vi "Recreate Client.vi"(8 "error in":errorcluster, 10 "cluster id":string, 11 "grpc client id in":T1) -> (0 "error out":errorcluster, 3 "grpc client id out":T1)   [LabVIEW 2020, in "Measurement Plugin Session Management V1.lvlib" / "Session Reservation.lvclass"]
uses:
  Session Reservation.lvclass
  <vilib>/gRPC/LabVIEW gRPC Library/Shared/grpcId.ctl
  Generated/Measurement Plugin Session Management Client/MeasurementLink Session Management Client.lvlib
  <vilib>/gRPC/LabVIEW gRPC Library/grpc-lvsupport-release.lvlib
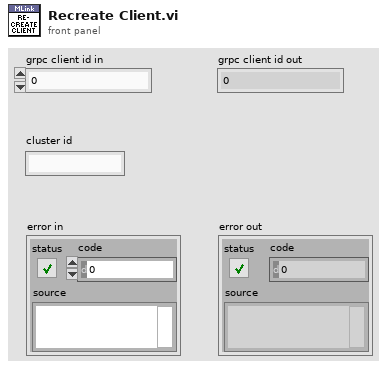
[diagram p1: front panel]
types:
  T1 = typedef "grpc-lvsupport-release.lvlib/grpcId.ctl" = u64
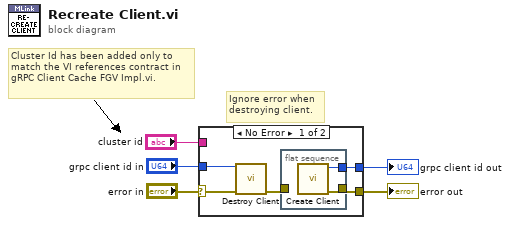
[diagram p0: block diagram]
diagram:
  # "Cluster Id has been added only to match the VI references contract in gRPC Client Cache FGV Impl.vi."
  # "Ignore error when\ndestroying client."
  n1 = case shown="No Error" "error in" {
    selector: "error in" -> [w9 w13]
    tunnel: [w8 w13] -> w4
    tunnel: [w7 _] -> w3
    tunnel: "grpc client id in" -> [w6 _]
    tunnel: "cluster id" -> [_ _]
    frame No Error {
      n2 = call "Destroy Client.vi"("error in"=w9, "gRPC ID"=w6) -> ("error out"=w10:errorcluster)  [unwired: 9 in]
      n3 = flat-sequence {
        tunnel: w10 -> [_]
        tunnel: [w12] -> w8
        tunnel: [w11] -> w7
        frame #0 {
          n4 = call "Create Client.vi"() -> ("error out"=w12:errorcluster, "grpc client id"=w11:T1)  [unwired: 10 in]
        }
      }
    }
    frame Error {
    }
  }
  "error out" <- w4
  "grpc client id out" <- w3
